vi "SR_Temperaturmessung_Simulation_2Kanal_work.vi"() -> ()   [LabVIEW 2020]
uses:
  Instance           3 35Saved   SR_Temperaturmessung_2Kanal .vi
  Instance           2 35Saved   SR_Temperaturmessung_2Kanal .vi
panel:
  out "Temperaturvergleich [°C]":dynamicdata(graph)
  out "T_Pt100 [°C]":dynamicdata(graph)
  out "U_Pt100 [V]":dynamicdata(graph)
  out "Messzeit [s]":dbl
  out "T_Termoelement [°C]":dynamicdata(graph)
  in  "Dateiheader":string[](array[string])=["Name(n): ", "Laborübung: Temperaturmessung", "Datum: xxx", "Messdatei: xxx.vi"]
  in  "Messung STOPP":bool
  in  "Spaltenüberschriften":string[](array[string])=["Zeit [s]", "U_Thermoelement [V]", "U_Pt100  [V]", "T_Thermoelement [°C]", "T_Pt100 [°C]"]
  out "dt":dbl
  in  "Messfrequenz":dbl=10.0
  in  "Format-String für EXCEL":string="%f\t%f\t%f\t%f\t%f\n"
  in  "Dateipfad (Dialog verwenden)":path=path "C:/Users/Messlabor_Kustos/Desktop/test.xls"
  in  "Operation (0:Öffnen)":T1(ring)=enum."replace or create"
  in  "Zugriff (0:Lesen/Schreiben)":enum16{"read/write", "read-only", "write-only"}(ring)=enum."write-only"
  out "U_Termoelement [V]":dynamicdata(graph)
  # "Dateioptionen"
  # "Spaltenbezeichnung im EXCEL-File"
  # "Messparameter"
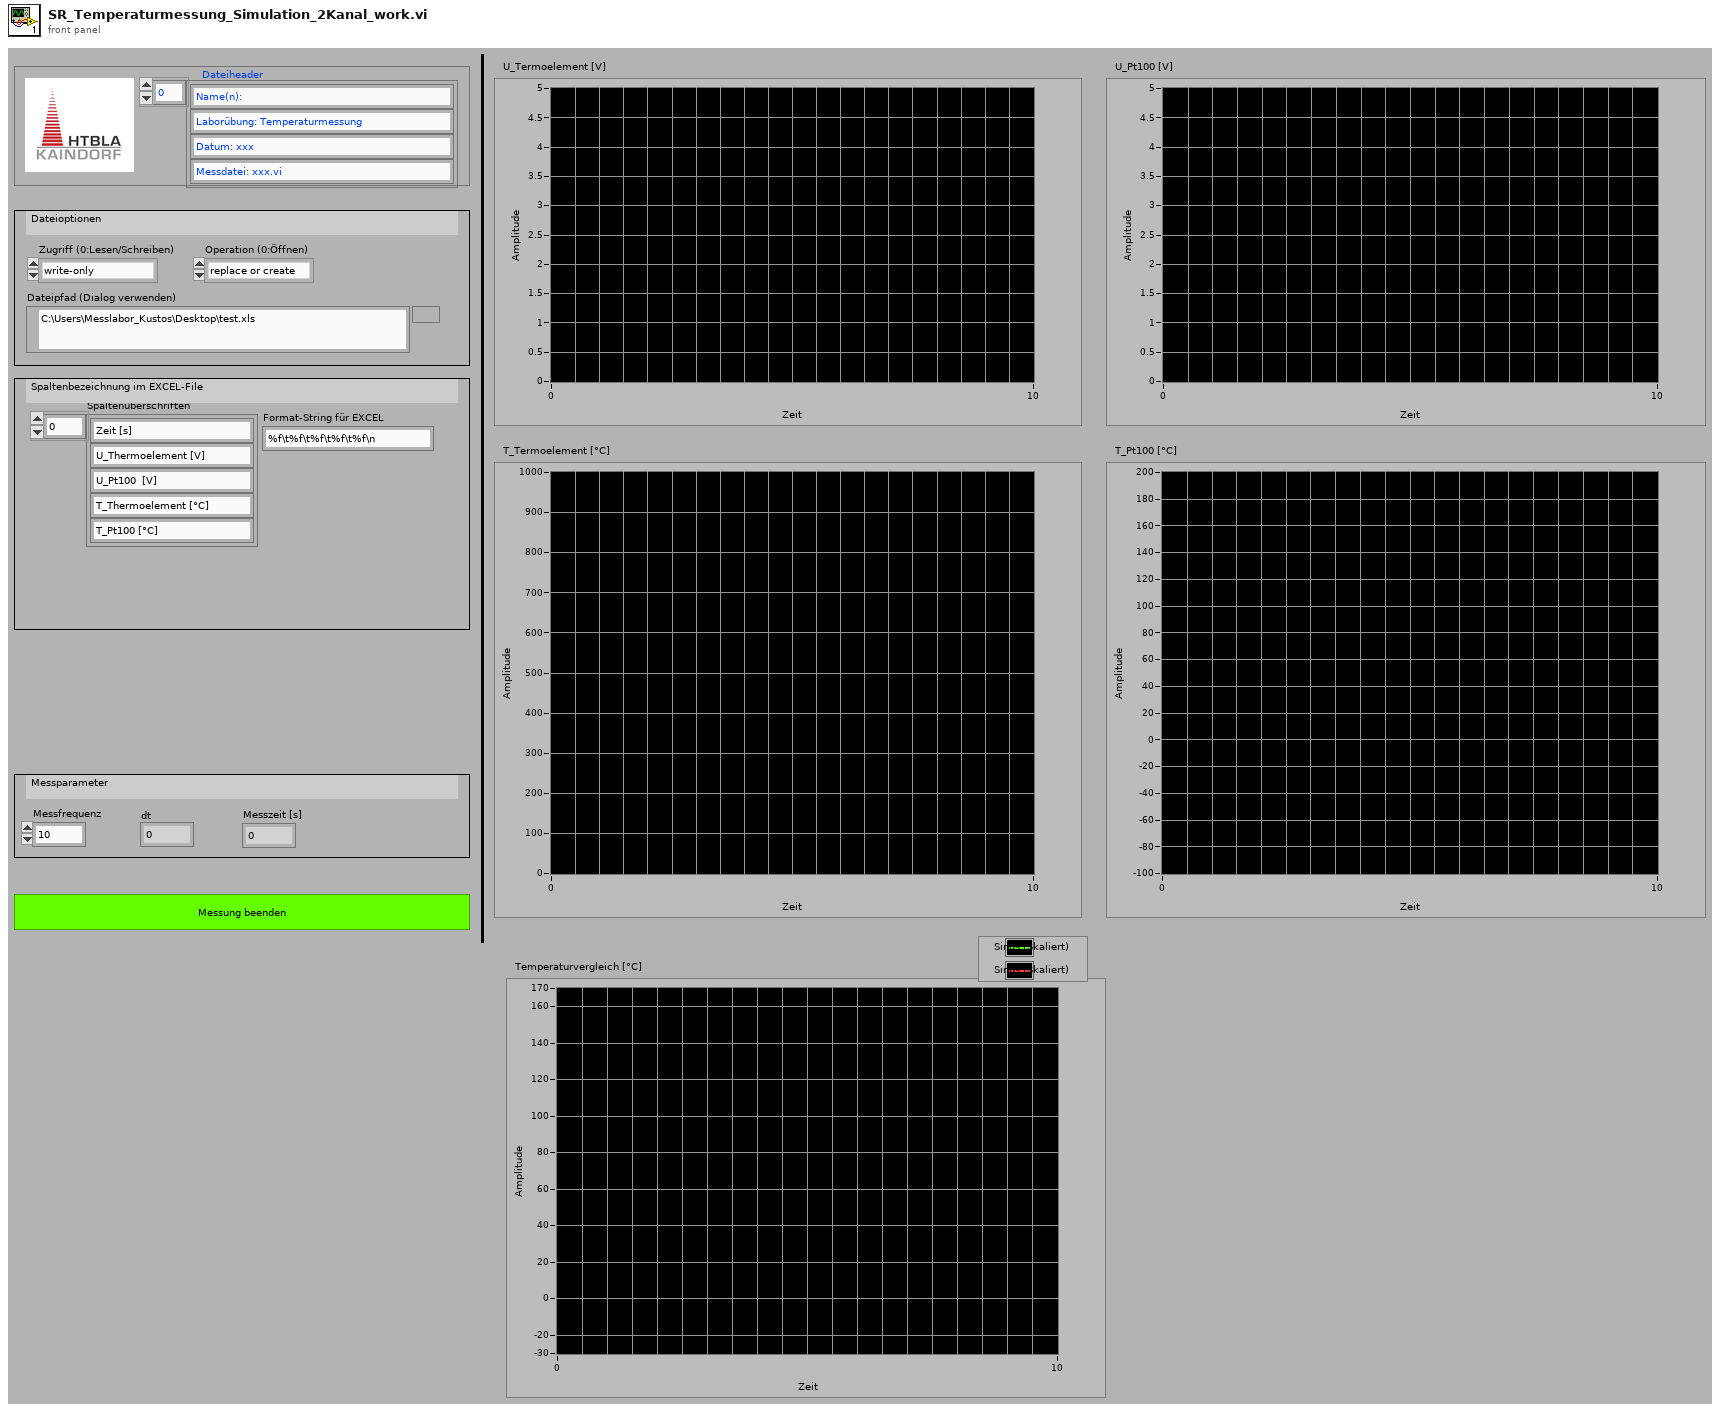
[diagram p1: front panel]
types:
  T1 = enum16{"open", "replace", "create", "open or create", "replace or create", "replace or create with confirmation"}
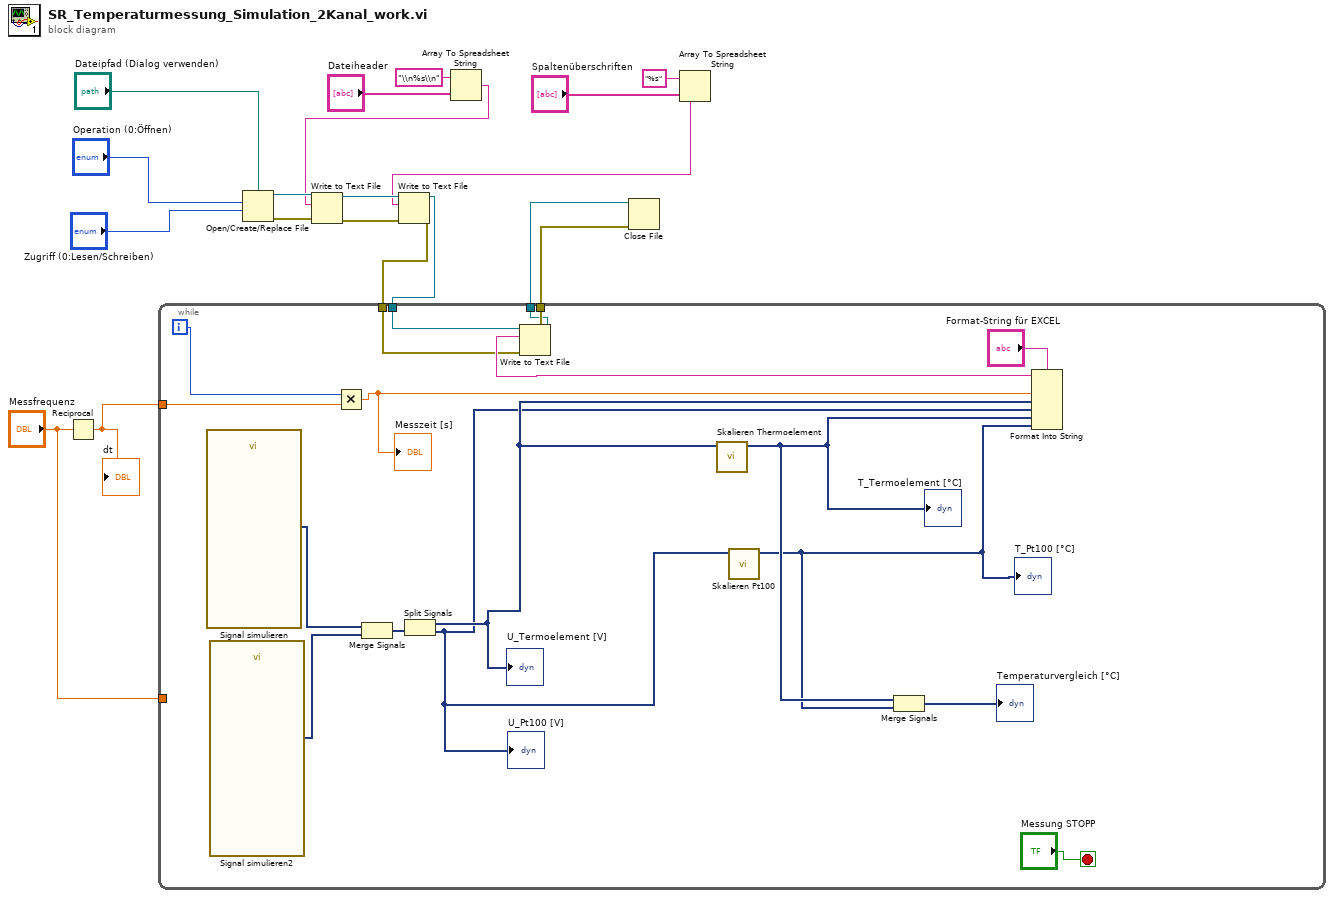
[diagram p0: block diagram]
diagram:
  n1 = Reciprocal(x="Messfrequenz") -> (1/x=w14:dbl)
  "dt" <- w14
  n2 = Open/Create/Replace File(file path (use dialog)="Dateipfad (Dialog verwenden)", operation (0:open)="Operation (0:Öffnen)", access (0:read/write)="Zugriff (0:Lesen/Schreiben)") -> (refnum out=w13:refnum<file>, error out=w12:errorcluster)  [unwired: 3 in, 1 out]
  n3 = Array To Spreadsheet String(array="Dateiheader", 3:"\\n%s\\n" ("Format-String")) -> (spreadsheet string=w2:string)  [unwired: 1 in]
  n4 = Write to Text File(file (use dialog)=w13, text=w2, error in=w12) -> (refnum out=w7:refnum<file>, error out=w5:errorcluster)  [unwired: 1 in, 1 out]
  n5 = Array To Spreadsheet String(array="Spaltenüberschriften", 3:"%s" ("Format-String")) -> (spreadsheet string=w3:string)  [unwired: 1 in]
  n6 = Write to Text File(file (use dialog)=w7, text=w3, error in=w5) -> (refnum out=w6:refnum<file>, error out=w4:errorcluster)  [unwired: 1 in, 1 out]
  n7 = while {
    tunnel: [w37] -> w16
    tunnel: [w36] -> w15
    tunnel: w14 -> [w23]
    tunnel: w6 -> [w32]
    tunnel: w4 -> [w31]
    tunnel: "Messfrequenz" -> [_]
    i -> [w33]
    stop <- "Messung STOPP" stop-if-true
    n8 = call "Signal simulieren"() -> ("Sinus"=w21:dynamicdata)  [unwired: 14 in, 1 out]
    n9 = call "Signal simulieren2"() -> ("Sinus"=w20:dynamicdata)  [unwired: 14 in, 1 out]
    n10 = Multiply(x=w33, y=w23) -> (x*y=w29:dbl)
    "Messzeit [s]" <- w29
    n11 = Merge Signals(w21, w20) -> (w22:dynamicdata)
    n12 = Split Signals(w22) -> (w28:dynamicdata, w27:dynamicdata)  [unwired: 2 in]
    "U_Termoelement [V]" <- w28
    "U_Pt100 [V]" <- w27
    n13 = call "Skalieren Thermoelement"("Signals"=w28) -> ("Scaled Signals"=w26:dynamicdata)  [unwired: 9 in, 1 out]
    "T_Termoelement [°C]" <- w26
    n14 = call "Skalieren Pt100"("Signals"=w27) -> ("Scaled Signals"=w25:dynamicdata)  [unwired: 9 in, 1 out]
    "T_Pt100 [°C]" <- w25
    n15 = Merge Signals(w26, w25) -> (→"Temperaturvergleich [°C]":dynamicdata)
    n16 = Format Into String(format string="Format-String für EXCEL", w29, w28, w27, w26, w25) -> (resulting string=w34:string)  [unwired: 2 in, 1 out]
    n17 = Write to Text File(file (use dialog)=w32, text=w34, error in=w31) -> (refnum out=w36:refnum<file>, error out=w37:errorcluster)  [unwired: 1 in, 1 out]
  }
  n18 = Close File(refnum=w15, error in=w16) -> ()  [unwired: 2 out]
